vi "SetRF.vi"(0 "reference in":refnum<class "niMmWave_Transceiver.lvclass">, 5 "Port":string(combo), 7 "Frequency":dbl format="%#_6pHz", 9 "Gain":dbl format="%#_6fdb", 11 "error in (no error)":errorcluster) -> (4 "reference out":refnum<class "niMmWave_Transceiver.lvclass">, 15 "error out":errorcluster)   [LabVIEW 2019, in "niMmWave_Transceiver.lvclass"]
doc: "Set RF configuration for port:\nGain and frequency"
uses:
  niMmWave_Transceiver.lvclass
  mmWave HW Control/LO sources.ctl
  mmWave HW Control/LO export.ctl
  mmWave HW Control/mmWave HW Control.lvlib
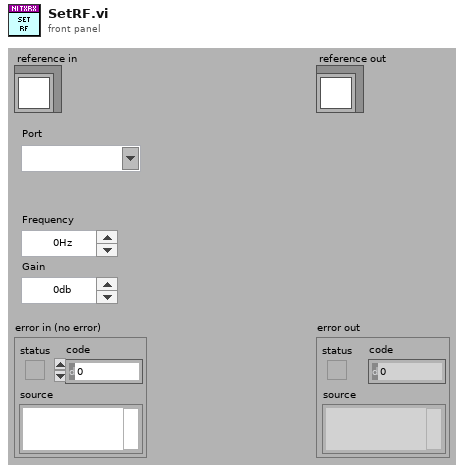
[diagram p1: front panel]
types:
  T1 = typedef "niMmWave_Transceiver.lvclass/ObjectAttributesRef.ctl" = refnum<data-value>
  T2 = typedef "niMmWave_Transceiver.lvclass/ObjectAttributes.ctl" = cluster{"session":T3[], "HW.RX resources":T17, "RF config":T18, "RX trigger options":T19, "TX trigger options":T19, "RX samples":i32, "Downloaded Bursts":map{string, T22}, "TX Fs":dbl, "RX Fs":dbl, "burst sequence":string[]}
  T3 = typedef "Session.ctl" = cluster{"3620 session":refnum<queue>, "tx baseband session":T4, "rx baseband session":T12, "tx gain (dB)":dbl, "rx gain (dB)":dbl, "hardware configuration":T13, "gain ranging":T15[], "pxi trigger bus information":T16}
  T4 = typedef "Tx Baseband Session.ctl" = cluster{"3610 session":T5, "7902 reference":T11}
  T5 = typedef "ni3610_and_ni3630_Driver_Lib.lvlib/Main Settings.ctl" = cluster{"VISA resource name":refnum<visa-resource-name>, "Address Space":T6, "window_offset":u32, "register_addresses":T7, "required_MM_fpga_version":cluster{"signature":u32, "hardware":u32, "current revision":u32, "oldest revision":u32}, "CPLD Oldest Compat Version ":cluster{"hardware":u32, "CPLD firmware":u32}, "MM_FPGA_image_location":string, "is_init":bool, "card_type":T8, "DacLmkConfigFileName":string, "AdcLmkConfigFileName":string, "AdcConfigFileName":string, "DacConfigFileName_RevA":string, "DacConfigFileName_RevB":string, "Mulde hardware revision":u8, "bypass DAC PLL\n":bool, "IQ Card Revision":T9, "board capability":T10}
  T6 = typedef "VISA Register Access Address Space.ctl" = u16
  T7 = typedef "ni3610_and_ni3630_Driver_Lib.lvlib/Register Adresses.ctl" = cluster{"MM based Registers":cluster{"Revision":u32, "OldestCompatRev":u32, "signature":u32, "scratch":u32, "LedControl":u32, "BoardHwRev":u32, "BoardControl":u32, "ThermalStatus":u32, "BasebandStatus":u32, "BasebandControl":u32, "BasebandAuxSetup":u32, "BasebandAuxStatus":u32, "LmkSyncOutSetup":u32, " AdcSyncOutSetup":u32, " InjSyncOutSetup":u32, " PxiTrig0OutSetup":u32, " PxiTrig1OutSetup":u32, " PxiTrig2OutSetup":u32, " PxiTrig3OutSetup":u32, " PxiTrig4OutSetup":u32, " PxiTrig5OutSetup":u32, " PxiTrig6OutSetup":u32, " PxiTrig7OutSetup":u32}, "CPLD based Registers":cluster{"SlaveSignature":u32, "SlaveRevision":u32, "SlaveOldestCompatRev":u32, "SlaveScratch":u32, "SlaveSetup":u32, "SlaveStatus":u32, "IDacReg_offset":u32, "LMKRegGrp0_offset":u32, "QDacReg_offset":u32, "BrdTempSensorVal":u32, "TempSensorPowerDown":u32, "GPIOReg_offset":u32, "IAdcReg_offset":u32, "QAdcReg_offset":u32, "LMKRegGrp1_offset":u32, "QadcTempSensorVal":u32, "IadcTempSensorVal":u32, "RevisionReg":u32, "VcxoReg":u32, "CpldStatusReg":u32, "PowerReg":u32, "VBiasEnReg":u32, "ExtRefOeReg":u32, "QdacCtrlReg":u32, "QdacStatusReg":u32, "IdacCtrlReg":u32, "IdacStatusReg":u32, "QdacJtagIn":u32, "QdacJtagOut":u32, "IdacJtagIn":u32, "IdacJtagOut":u32, "IqDcSetupReg":u32, "QadcStatusReg":u32, "IadcStatusReg":u32, "BrdSetupReg":u32, "IqDcRevisionReg":u32, "PllStatusReg":u32, "EndpointScratchReg":u32, "AdcSyncCfgReg":u32, "IqCardOpampReg":u32}, "CPLD Register Offset":u32, "MM  Register Offset":u32, " PxiTrig0OutSetup":u32}
  T8 = typedef "ni3610_and_ni3630_Driver_Lib.lvlib/Base Card Type.ctl" = enum16{"unspecified", "ADC", "DAC"}
  T9 = typedef "ni3610_and_ni3630_Driver_Lib.lvlib/IQ Card Revision.ctl" = enum16{"RevA", "RevB", "RevC", "RevD"}
  T10 = typedef "ni3610_and_ni3630_Driver_Lib.lvlib/Board Capability.ctl" = cluster{"baseband sync":enum16{"no baseband sync", "baseband sync"}}
  T11 = typedef "Blank FPGA Reference.ctl" = refnum<k20>
  T12 = typedef "Rx Baseband Session.ctl" = cluster{"3630 session":T5, "7902 reference":T11}
  T13 = typedef "Hardware Configuration.ctl" = cluster{"direction":T14, "baseband only":bool}
  T14 = typedef "Direction.ctl" = enum16{"Transceiver", "Receiver", "Transmitter"}
  T15 = typedef "Gain Ranging.ctl" = cluster{"gain ranging active scope":string, "gain ranging stream session":refnum<k20>}
  T16 = typedef "PXI Trigger Bus Info.ctl" = cluster{"chassis resource name":refnum<visa-resource-name>, "7902R (TX)":i16, "3610 (TX)":i16, "3620 (IF)":i16, "3630 (RX)":i16, "7902R (RX)":i16}
  T17 = typedef "mmWave HW Control.lvlib/HW TXRX resources cluster.ctl" = cluster{"TX_DAC":refnum<visa-resource-name>, "TX_FPGA":tag, "IF":tag, "RX_ADC":refnum<visa-resource-name>, "RX_FPGA":tag}
  T18 = typedef "mmWave HW Control.lvlib/HW TXRX RF config cluster.ctl" = cluster{"TX.Frequency":dbl, "TX.Gain":dbl, "TX.mmWave adapter":string, "RX.Frequency":dbl, "RX.Gain":dbl, "RX.mmWave adapter":string}
  T19 = typedef "TX trigger config.ctl" = cluster{"delay":dbl, "trig source":T20, "PXI src":i32, "export":T21, "PXI dest":i32}
  T20 = typedef "FPGA Utility.lvlib/FPGA driver trigger source.ctl" = enum16{"Use Tclk", "PXI_Trig", "Aurora RX trig"}
  T21 = typedef "FPGA Utility.lvlib/FPGA driver trigger destination.ctl" = enum16{"None", "Source trig", "Synced trig", "Delayed sync"}
  T22 = typedef "niMmWave_Transceiver.lvclass/BurstInfo.ctl" = cluster{"starting addr":u32, "end addr":u32}
  T23 = typedef "mmWave HW Control.lvlib/LO export.ctl" = cluster{"TX LO1 export":bool, "TX LO1 export level":dbl, "RX LO1 export":bool, "RX LO1 export level":dbl, "LO2 export":bool, "LO2 export level":dbl}
  T24 = typedef "mmWave HW Control.lvlib/LO sources.ctl" = cluster{"RX/LO1 src":string, "TX/LO1 src":string, "LO2 src":string}
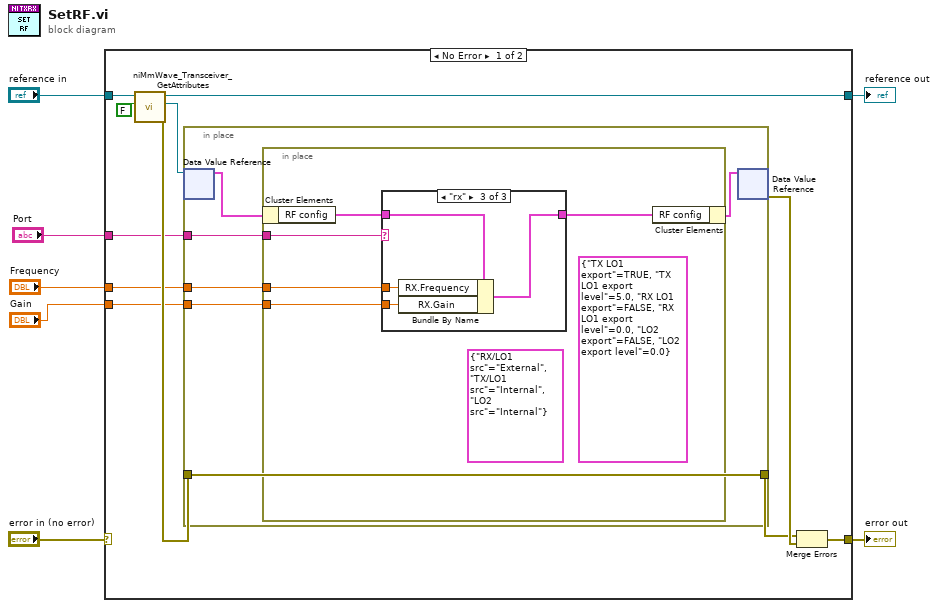
[diagram p0: block diagram]
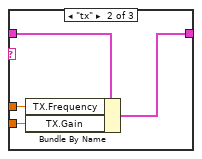
[diagram p3: hidden frame]
diagram:
  n1 = case shown="No Error" "error in (no error)" {
    selector: "error in (no error)" -> [_ w40]
    tunnel: [w18 w40] -> w6
    tunnel: [w12 w39] -> w4
    tunnel: "reference in" -> [w15 w39]
    tunnel: "Port" -> [w10 _]
    tunnel: "Frequency" -> [w9 _]
    tunnel: "Gain" -> [w8 _]
    frame No Error {
      n2 = call "niMmWave_Transceiver_GetAttributes.vi"("return data? (T)"=FALSE, "reference in"=w15) -> ("error out"=w13:errorcluster, "attributes ref"=w11:T1, "reference out"=w12:refnum<class "niMmWave_Transceiver.lvclass">)  [unwired: 6 in, 1 out]
      n3 = in-place {
        in-place-border: w13 -> [w22]
        in-place-border: [w22] -> w16
        in-place-border: w10 -> [w21]
        in-place-border: w9 -> [w20]
        in-place-border: w8 -> [w19]
        n4 = in-place-dvr #1(w11) -> (w23:T2)  [unwired: 1 out]
        n5 = in-place {
          in-place-border: w21 -> [w27]
          in-place-border: w20 -> [w26]
          in-place-border: w19 -> [w25]
          (unwired) T23 {"TX LO1 export"=TRUE, "TX LO1 export level"=5.0, "RX LO1 export"=FALSE, "RX LO1 export level"=0.0, "LO2 export"=FALSE, "LO2 export level"=0.0} ("LO Export")
          (unwired) T24 {"RX/LO1 src"="External", "TX/LO1 src"="Internal", "LO2 src"="Internal"} ("LO sources")
          n6 = in-place-cluster #2(w23) -> ("RF config"=w28:T18)
          n7 = case shown="\"rx\"" w27 {
            tunnel: [w30 w33 w37] -> w29
            tunnel: w28 -> [w30 w34 w38]
            tunnel: w26 -> [_ w32 w36]
            tunnel: w25 -> [_ w31 w35]
            frame "False", Default {
            }
            frame "tx" {
              n8 = Bundle By Name(cluster=w34, "TX.Frequency"=w32, "TX.Gain"=w31) -> (w33:T18)
            }
            frame "rx" {
              n9 = Bundle By Name(cluster=w38, "RX.Frequency"=w36, "RX.Gain"=w35) -> (w37:T18)
            }
          }
          n10 = in-place-cluster #2("RF config"=w29) -> (w24:T2)
        }
        n11 = in-place-dvr #1(w24) -> (w17:errorcluster)  [unwired: 1 out]
      }
      n12 = Merge Errors(w16, w17) -> (w18:errorcluster)
    }
    frame Error {
    }
  }
  "error out" <- w6
  "reference out" <- w4
